vi "Add_Shortcut.vi"(8 "error in (no error)":errorcluster, 10 "new shortcut":T1, 11 "Installer in":refnum<class "Installer.lvclass">) -> (0 "error out":errorcluster, 3 "Installer out":refnum<class "Installer.lvclass">)   [LabVIEW 2020, in "Installer.lvclass"]
uses:
  <vilib>/AppBuilder/IB_Classes/Installer/Installer.lvclass
  <vilib>/AppBuilder/IB_Classes/Installer/Installer.lvclass/Installer.ctl
  <resource>/Framework/Providers/Builds/Installer/CDK_sTypeDef_ShortcutAddress.ctl
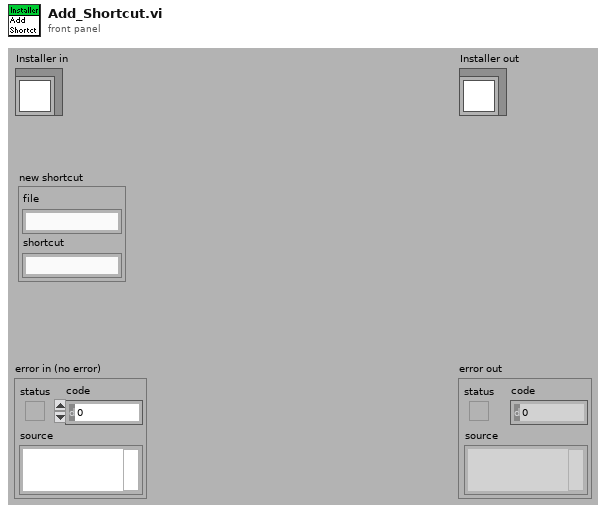
[diagram p1: front panel]
types:
  T1 = typedef "CDK_sTypeDef_ShortcutAddress.ctl" = cluster{"file":string, "shortcut":string}
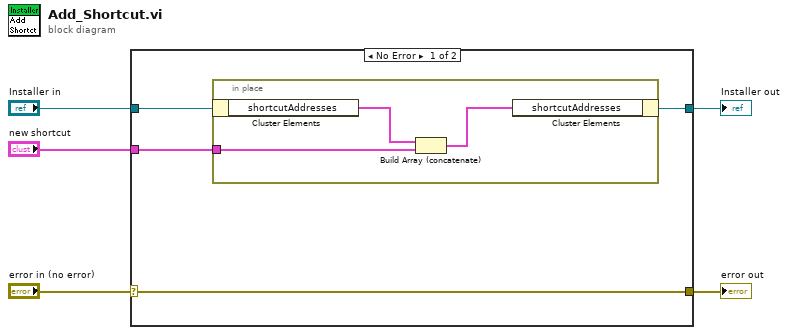
[diagram p0: block diagram]
diagram:
  n1 = case shown="No Error" "error in (no error)" {
    selector: "error in (no error)" -> [w9 w14]
    tunnel: [w9 w14] -> w4
    tunnel: [w6 w13] -> w2
    tunnel: "Installer in" -> [w7 w13]
    tunnel: "new shortcut" -> [w8 _]
    frame No Error {
      n2 = in-place {
        in-place-border: w8 -> [w10]
        n3 = in-place-cluster #1(w7) -> ("shortcutAddresses"=w12:T1[])
        n4 = Build Array (concatenate)(w12, w10) -> (w11:T1[])
        n5 = in-place-cluster #1("shortcutAddresses"=w11) -> (w6:refnum<class "Installer.lvclass">)
      }
    }
    frame Error {
    }
  }
  "error out" <- w4
  "Installer out" <- w2
